vi "Message_VI.vi"() -> ()   [LabVIEW 2010]
panel:
  in  "stop":bool
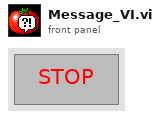
[diagram p1: front panel]
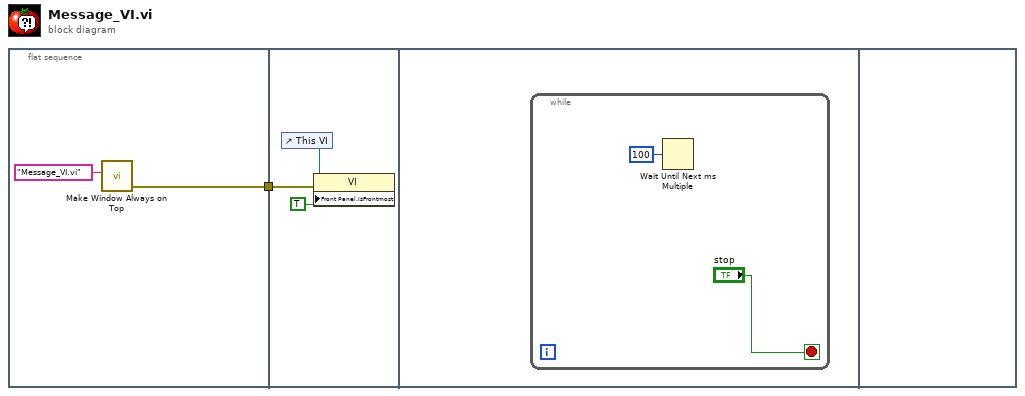
[diagram p0: block diagram]
diagram:
  n1 = flat-sequence {
    tunnel: [w2] -> w1
    tunnel: w1 -> [w4]
    frame #0 {
      n2 = call "Make Window Always on Top.vi"("window name (\"\")"="Message_VI.vi" ("window name (\"\")")) -> ("error out"=w2:errorcluster)  [unwired: 5 in, 1 out]
    }
    frame #1 {
      n3 = control-ref of="This VI"() -> (w6:refnum<vi>)
      n4 = property class="VI"(reference=w6, error in=w4, "Front Panel.IsFrontmost"=TRUE ("Front Panel Window:Is Frontmost")) -> ()  [unwired: 2 out]
    }
    frame #2 {
      n5 = while {
        stop <- "stop" stop-if-true
        n6 = Wait Until Next ms Multiple(millisecond multiple=u32 100) -> ()  [unwired: 1 out]
      }
    }
    frame #3 {
    }
  }
